vi "LEBITVacuum.SetPLC.vi"(0 "i ref in":refnum<vi>, 1 "CommandName":string, 2 "index of element":i32, 3 "Value":i16, 4 "log?":bool, 5 "error IO":errorcluster) -> (14 "i ref out":refnum<vi>, 19 "error out":errorcluster)   [LabVIEW 2014, in "LEBITVacuum.lvlib"]
uses:
  LEBITVacuum.lvlib
  CS_Core/CSSystem/CoreDefs/CoreDefs.error_type.ctl
  CS_Core/CSSystem/CoreDefs/CoreDefs.error_severity.ctl
  CS_Core/CSSystem/CoreLib/CoreLib.lvlib
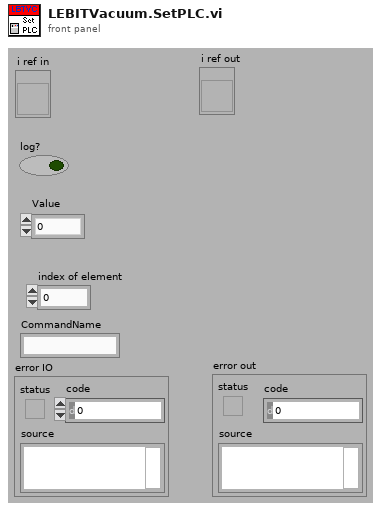
[diagram p1: front panel]
types:
  T1 = typedef "CoreDefs.error_severity.ctl" = enum16{"undefined", "information", "warning", "error", "fatal"}
  T2 = typedef "CoreDefs.error_type.ctl" = enum16{"no error", "can't load process", "can't unload process", "process does not exist", "can't install process", "can't remove process", "unknown function", "time out", "can't execute function", "duplicate queue name", "super not found", "caller queue invalid", "can't ping process", "unknown error", "VISA Error", "VISA timeout", "GPIB timeout", "GPIB error", "communication error", "data type mismatch", "can't read data from OPC server", "can't write data to OPC server", "OET error", "function not implemented", "process already exists", "invalid Shared Variable name", "error writing Shared Variable", "error reading Shared Variable", "invalid client name", "corrupt database", "unknown class", "call not authorized", "parameter out of range", "OET timeout: can't get data to modify", "invalid queue name", "requested operation incompatible with current state", "event undefined", "event disabled", "state undefined", "caller is not a friend", "EventBuilder: bad eventID", "EventBuilder: no DAQ devices", "a thread must not stop itself", "UNUSED ELEMENT4", "DiscArchiver: eventData incomplete", "DiscArchiver: eventData does not belong to run", "DiscArchiver: can't open file", "DiscArchiver: can't write to file", "DiscArchiver: available disc space low", "can't acquire semaphore", "error reading data from database", "notifier object is not existing", "can't register process", "can't unregister process", "illegal event type", "object disabled", "object already exists", "can't change state", "Instrument not found", "no connection to remote node", "invalid reference", "N/A", "UNUSED ELEMENT 1", "element not found", "illegal TCP/IP connection detected", "object does not exist", "invalid access ID", "unknown CS system", "invalid privilige", "unsupported data type", "unsupported server type", "IO server already exists", "Shared Variable already exists"}
  T3 = typedef "LEBITVacuum.lvlib/LEBITVacuum.i attribute.ctl" = cluster{"setValuePLC":string[], "nickNames":string[], "setValuePLCServiceID":i32[], "monValuePLC":string[], "SetValueServiceID":i32[], "MonValueServiceID":i32[], "SetValue":i16[], "AllPLCValues":string[], "CondSpecial2DArray":string[][], "CondSpecialIndex":i32[], "ReasonForLocking":string, "ReasonForLockingID":i32, "enableValuePLC":string[], "OverwriteCloseSafetyPLC":string[], "OverwriteOpenSafetyPLC":string[], "OverwriteCloseSafetyPLCServiceID":i32[], "OverwriteOpenSafetyPLCServiceID":i32[], "MKS Address Array":i32[][], "MKS MeasurementServiceID":i32[], "MKS Measurement":string[], "CRYO Measurement":string[][], "CRYO MeasurementServiceID":i32[], "Special":string[], "Start Date":string, "MKS VISA resource":refnum<visa-resource-name>, "CRYO VISA resource":refnum<visa-resource-name>}
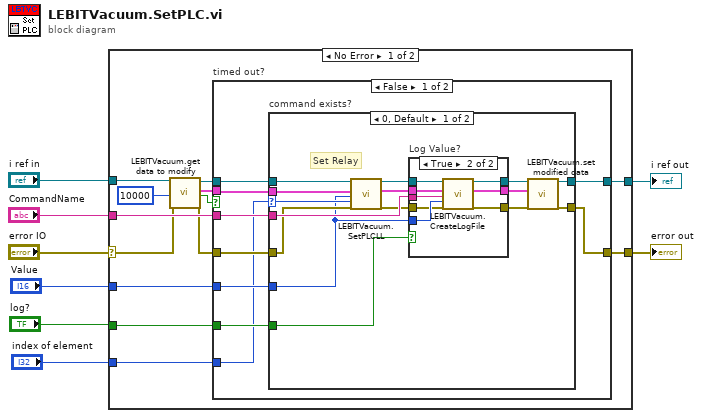
[diagram p0: block diagram]
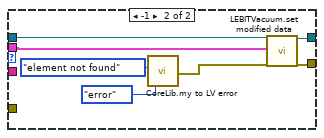
[diagram p3: hidden frame]
diagram:
  n1 = case shown="No Error" "error IO" {
    selector: "error IO" -> [w15 w66]
    tunnel: "CommandName" -> [w20 _]
    tunnel: "i ref in" -> [w18 w67]
    tunnel: [w17 w66] -> w6
    tunnel: [w16 w67] -> w5
    tunnel: "log?" -> [w11 _]
    tunnel: "Value" -> [w10 _]
    tunnel: "index of element" -> [w9 _]
    frame No Error {
      n2 = call "LEBITVacuum.get data to modify.vi"("i ref in"=w18, "ms timeout (10000)"=10000, "error in (no error)"=w15) -> ("i ref out"=w19:refnum<vi>, "i attribute"=w21:T3, "timed out"=w13:bool, "error out"=w12:errorcluster)  [unwired: 13 in]
      n3 = case "timed out?" shown="False" w13 {
        tunnel: w21 -> [w30 _]
        tunnel: w20 -> [w25 _]
        tunnel: w19 -> [w29 w65]
        tunnel: [w27 w64] -> w17
        tunnel: [w26 w65] -> w16
        tunnel: w12 -> [w28 w64]
        tunnel: w11 -> [w24 _]
        tunnel: w10 -> [w23 _]
        tunnel: w9 -> [w22 _]
        frame False {
          n4 = case "command exists?" shown="0, Default" w22 {
            selector: w22 -> [w32 _]
            tunnel: [w44 w60] -> w26
            tunnel: [w45 w57] -> w27
            tunnel: w29 -> [w35 w61]
            tunnel: w30 -> [w34 w59]
            tunnel: w28 -> [w33 _]
            tunnel: w25 -> [w43 _]
            tunnel: w24 -> [w42 _]
            tunnel: w23 -> [w31 _]
            frame 0, Default {
              # "Set Relay"
              n5 = call "LEBITVacuum.SetPLCLL.vi"("i ref in"=w35, "i attribute in"=w34, "SetValue"=w31, "index of element"=w32, "error IO"=w33) -> ("i ref out"=w40:refnum<vi>, "i attribute out"=w39:T3, "error out"=w41:errorcluster)  [unwired: 12 in]
              n6 = case "Log Value?" shown="True" w42 {
                tunnel: w43 -> [_ w56]
                tunnel: w31 -> [_ w55]
                tunnel: w41 -> [w48 w54]
                tunnel: [w48 w53] -> w37
                tunnel: w40 -> [w47 w51]
                tunnel: [w47 w52] -> w38
                tunnel: w39 -> [w46 w49]
                tunnel: [w46 w50] -> w36
                frame False {
                }
                frame True {
                  n7 = call "LEBITVacuum.CreateLogFile.vi"("i ref in"=w51, "i attribute in"=w49, "nickName"=w56, "value"=w55, "error in"=w54) -> ("i ref out"=w52:refnum<vi>, "i attribute out"=w50:T3, "error out"=w53:errorcluster)  [unwired: 12 in]
                }
              }
              n8 = call "LEBITVacuum.set modified data.vi"("i ref in"=w38, "i attribute"=w36, "error in (no error)"=w37) -> ("i ref out"=w44:refnum<vi>, "error out"=w45:errorcluster)  [unwired: 15 in]
            }
            frame -1 {
              n9 = call "CoreLib.my to LV error.vi"("ErrorTypes"=CoreDefs.error_type."element not found", "severityLevel"=CoreDefs.error_severity."error") -> ("myErrorCluster"=w58:errorcluster)  [unwired: 16 in, 1 out]
              n10 = call "LEBITVacuum.set modified data.vi"("i ref in"=w61, "i attribute"=w59, "error in (no error)"=w58) -> ("i ref out"=w60:refnum<vi>, "error out"=w57:errorcluster)  [unwired: 15 in]
            }
          }
        }
        frame True {
        }
      }
    }
    frame Error {
    }
  }
  "error out" <- w6
  "i ref out" <- w5
